vi "Start-stop asking for run cfg.vi"(8 "error in (no error)":errorcluster, 10 "Infinite Message Selector":T1, 11 "Guardian in":refnum<class "Guardian.lvclass">) -> (0 "error out":errorcluster, 3 "Guardian out":refnum<class "Guardian.lvclass">)   [LabVIEW 2026, in "TALOS.lvlib" / "Guardian.lvlib" / "Guardian.lvclass"]
uses:
  Guardian.lvclass
  Ancestor/Ancestor/Infinite Message Selector.ctl
  Guardian Messages/Ask for Run Config Msg/Ask for Run Config Msg.lvclass
  C:/LabVIEW Code/TALOS/builds/Actor Framework PPL/Actor Framework.lvlibp/1abvi3w/vi.lib/ActorFramework/Message/Message.lvclass
  Ancestor/Ancestor/Ancestor.lvclass
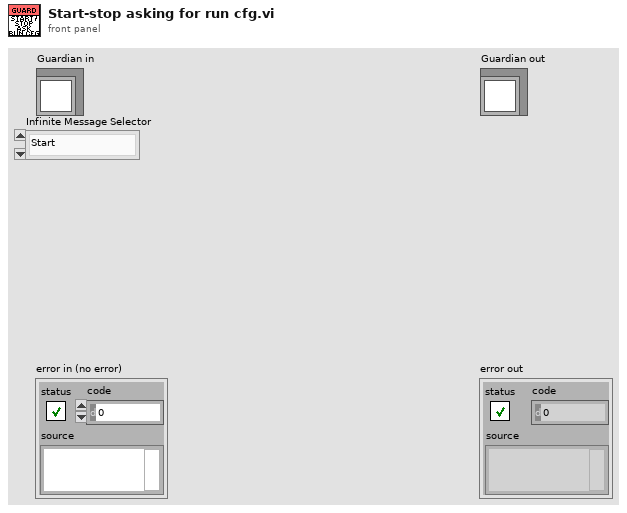
[diagram p1: front panel]
types:
  T1 = typedef "TALOS.lvlib/Ancestor.lvlib/Ancestor.lvclass/Infinite Message Selector.ctl" = enum16{"Start", "Stop", "Check", "Flush (Stop all)", "Init"}
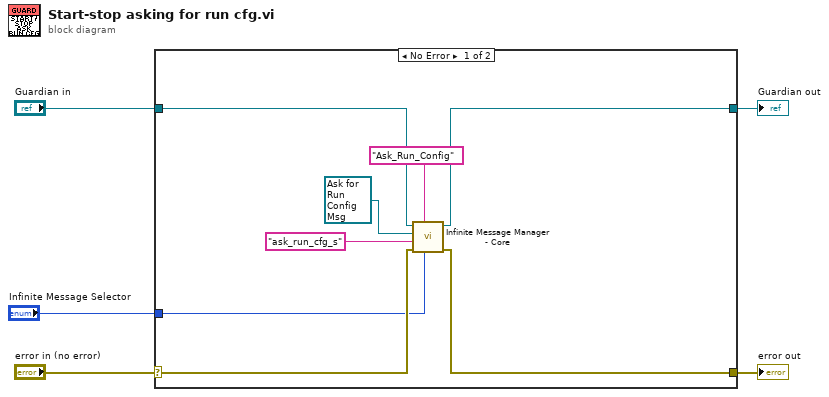
[diagram p0: block diagram]
diagram:
  n1 = case shown="No Error" "error in (no error)" {
    selector: "error in (no error)" -> [w11 w15]
    tunnel: [w10 w15] -> w4
    tunnel: [w13 w14] -> w2
    tunnel: "Guardian in" -> [w12 w14]
    tunnel: "Infinite Message Selector" -> [w8 _]
    frame No Error {
      n2 = call-dynamic "Infinite Message Manager - Core.vi"("Infinite Message Selector"=w8, "Msg ID"="Ask_Run_Config", "error in (no error)"=w11, "Tau parameter"="ask_run_cfg_s", "Actor Framework:Message"=refnum<class "Ask for Run Config Msg.lvclass"> refnum ("TALOS.lvlib:Guardian.lvlib:Ask for Run Config Msg.lvclass"), "Ancestor in"=w12) -> ("error out"=w10:errorcluster, "Ancestor out"=w13:refnum<class "Guardian.lvclass">)  [unwired: 3 in, 1 out]
    }
    frame Error {
    }
  }
  "error out" <- w4
  "Guardian out" <- w2
